vi "Day 05 Part 1.vi"(11 "Input":string) -> (3 "Output":i32)   [LabVIEW 2021]
panel:
  out "Intensity Graph":i32[][](graph)
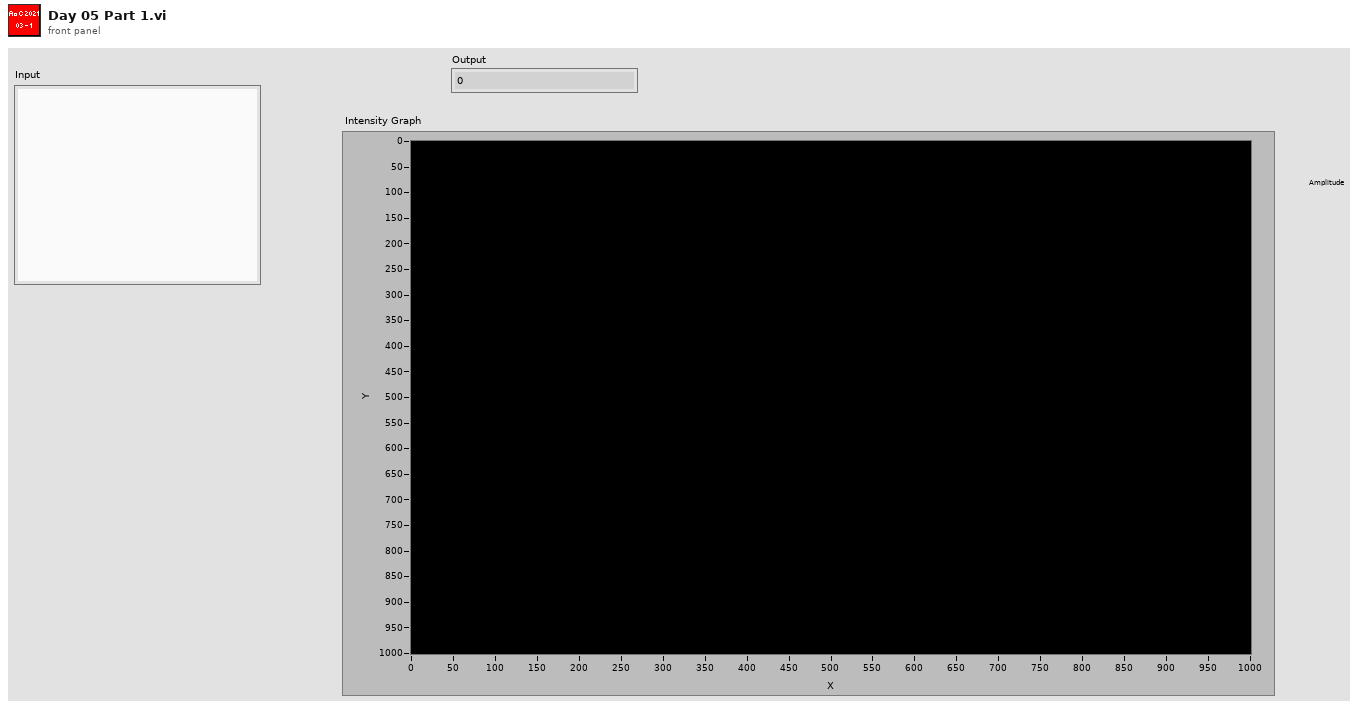
[diagram p1: front panel]
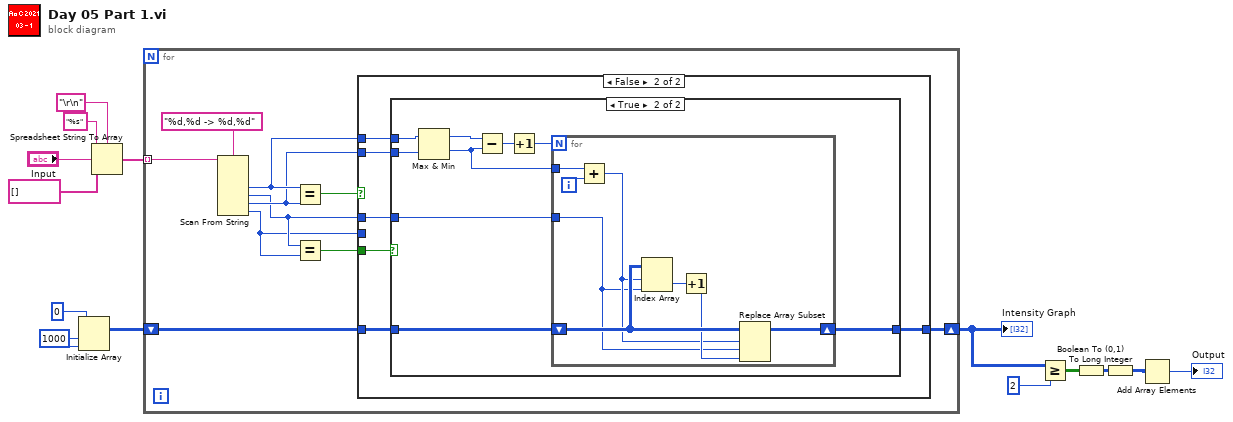
[diagram p0: block diagram]
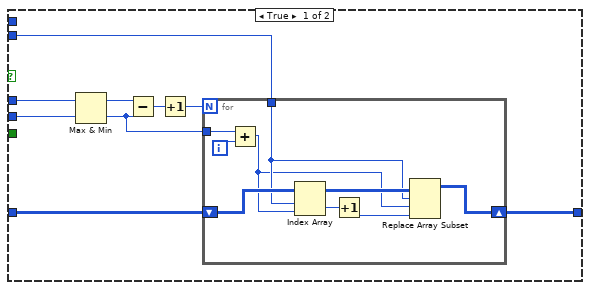
[diagram p2: hidden frame]
diagram:
  w9 = 1000 ("dimension size")
  n1 = Initialize Array(0, w9, w9) -> (w4:i32[][])
  n2 = Spreadsheet String To Array(delimiter (Tab)="\r\n", format string="%s", spreadsheet string="Input", array type (2D Dbl)=string[] []) -> (array=w10:string[])
  n3 = for {
    tunnel: w10 -> [w24] mode=indexing
    shift-right: [w15] -> w3
    shift-left: w4 -> [w16]
    n4 = Scan From String(format string="%d,%d -> %d,%d", input string=w24) -> (output 1=w22:i32, output 2=w20:i32, output 3=w21:i32, output 4=w19:i32)  [unwired: 6 in, 3 out]
    n5 = Equal?(x=w22, y=w21) -> (x = y?=w18:bool)
    n6 = Equal?(x=w20, y=w19) -> (x = y?=w17:bool)
    n7 = case shown="False" w18 {
      tunnel: w22 -> [_ w47]
      tunnel: w21 -> [w31 w46]
      tunnel: w20 -> [w30 w45]
      tunnel: w19 -> [w29 _]
      tunnel: w17 -> [_ w44]
      tunnel: w16 -> [w26 w43]
      tunnel: [w25 w42] -> w15
      frame True {
        n8 = Max & Min(x=w30, y=w29) -> (max(x,y)=w28:i32, min(x,y)=w27:i32)
        n9 = Subtract(x=w28, y=w27) -> (x-y=w33:i32)
        n10 = Increment(x=w33) -> (x+1=w32:i32)
        n11 = for {
          N: w32 -> [_]
          tunnel: w27 -> [w40]
          tunnel: w31 -> [w36]
          shift-right: [w34] -> w25
          shift-left: w26 -> [w38]
          i -> [w41]
          n12 = Add(x=w40, y=w41) -> (x+y=w35:i32)
          n13 = Index Array(array=w38, index (row)=w36, index (col)=w35) -> (element=w39:i32)
          n14 = Increment(x=w39) -> (x+1=w37:i32)
          n15 = Replace Array Subset(array=w38, new element=w37, index (row)=w36, index (col)=w35) -> (w34:i32[][])
        }
      }
      frame False {
        n16 = case shown="True" w44 {
          tunnel: w47 -> [_ w55]
          tunnel: w46 -> [_ w53]
          tunnel: w45 -> [_ w51]
          tunnel: w43 -> [w48 w50]
          tunnel: [w48 w49] -> w42
          frame False {
          }
          frame True {
            n17 = Max & Min(x=w55, y=w53) -> (max(x,y)=w54:i32, min(x,y)=w52:i32)
            n18 = Subtract(x=w54, y=w52) -> (x-y=w57:i32)
            n19 = Increment(x=w57) -> (x+1=w56:i32)
            n20 = for {
              N: w56 -> [_]
              tunnel: w52 -> [w64]
              tunnel: w51 -> [w59]
              shift-right: [w58] -> w49
              shift-left: w50 -> [w62]
              i -> [w65]
              n21 = Add(x=w64, y=w65) -> (x+y=w60:i32)
              n22 = Index Array(array=w62, index (row)=w60, index (col)=w59) -> (element=w63:i32)
              n23 = Increment(x=w63) -> (x+1=w61:i32)
              n24 = Replace Array Subset(array=w62, new element=w61, index (row)=w60, index (col)=w59) -> (w58:i32[][])
            }
          }
        }
      }
    }
  }
  "Intensity Graph" <- w3
  n25 = Greater Or Equal?(x=w3, y=2) -> (x >= y?=w6:bool[][])
  n26 = Boolean To (0,1)(Boolean=w6) -> (0, 1=w5:i16[][])
  n27 = To Long Integer(number=w5) -> (32bit integer=w1:i32[][])
  n28 = Add Array Elements(numeric array=w1) -> (sum=→"Output":i32)
